vi "ConvertDates.vi"(1 "Dates":string[](array[string])=["10/14/2011\u0000\u0000\u0000\u0000\u0000\u0000\u0000\u0000\u0000\u0000\u0000\u0000", "10/14/2011 11:14:43 PM", "10/14/2011 3:56:30 PM\u0000", "10/14/2011 4:18:24 PM\u0000", "10/15/2011\u0000\u0000\u0000\u0000\u0000\u0000\u0000\u0000\u0000\u0000\u0000\u0000", "10/15/2011 7:54:35 AM\u0000", "10/16/2011\u0000\u0000\u0000\u0000\u0000\u0000\u0000\u0000\u0000\u0000\u0000\u0000"]) -> (0 "ConvertedDates":string[](array[string]))   [LabVIEW 2012]
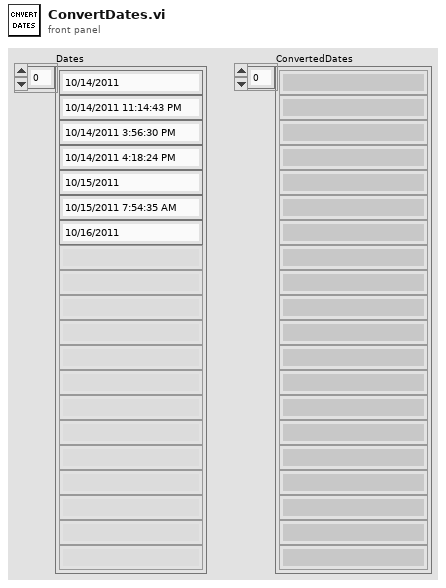
[diagram p1: front panel]
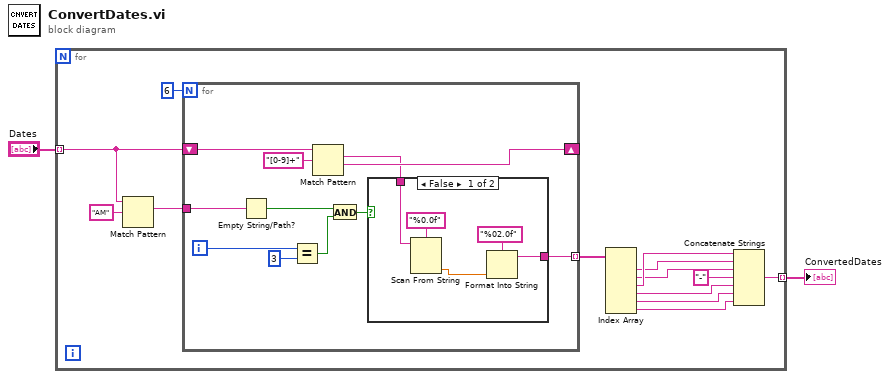
[diagram p0: block diagram]
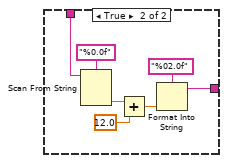
[diagram p2: hidden frame]
diagram:
  n1 = for {
    tunnel: "Dates" -> [w13] mode=indexing
    tunnel: [w5] -> w1 mode=indexing
    n2 = Match Pattern(string=w13, regular expression="AM") -> (match substring=w12:string)  [unwired: 1 in, 3 out]
    n3 = for {
      N: 6 -> [_]
      shift-right: [w25] -> _
      shift-left: w13 -> [w24]
      tunnel: w12 -> [w20]
      tunnel: [w16] -> w11 mode=indexing
      i -> [w23]
      n4 = Empty String/Path?(string/path=w20) -> (empty?=w19:bool)
      n5 = Equal?(x=w23, y=3) -> (x = y?=w21:bool)
      n6 = Match Pattern(string=w24, regular expression="[0-9]+") -> (match substring=w17:string, after substring=w25:string)  [unwired: 1 in, 2 out]
      n7 = And(x=w19, y=w21) -> (x .and. y?=w18:bool)
      n8 = case shown="False" w18 {
        tunnel: w17 -> [w29 w38]
        tunnel: [w27 w33] -> w16
        frame False {
          n9 = Scan From String(format string="%0.0f", input string=w29) -> (output 1=w28:dbl)  [unwired: 3 in, 3 out]
          n10 = Format Into String(format string="%02.0f", w28) -> (resulting string=w27:string)  [unwired: 2 in, 1 out]
        }
        frame True {
          n11 = Scan From String(format string="%0.0f", input string=w38) -> (output 1=w37:dbl)  [unwired: 3 in, 3 out]
          n12 = Add(x=w37, y=12.0) -> (x+y=w35:dbl)
          n13 = Format Into String(format string="%02.0f", w35) -> (resulting string=w33:string)  [unwired: 2 in, 1 out]
        }
      }
    }
    n14 = Index Array(array=w11) -> (element #1=w4:string, element #2=w3:string, element #3=w10:string, element #4=w8:string, element #5=w7:string, element #6=w6:string)  [unwired: 6 in]
    n15 = Concatenate Strings(w10, w4, w3, "-" ("string"), w8, w7, w6) -> (w5:string)
  }
  "ConvertedDates" <- w1
